vi "Tosca-Stream AI Data.vi"(0 "state in":T1, 5 "Data":cluster{dbl[][], bool[][]}, 11 "error in (no error)":errorcluster, 13 "stream":T2) -> (4 "state out":T1, 8 "filename":string, 15 "error out":errorcluster)   [LabVIEW 2020]
uses:
  Typedefs/Tosca-AI Stream Controls.ctl
  Typedefs/Tosca-AI Plot State.ctl
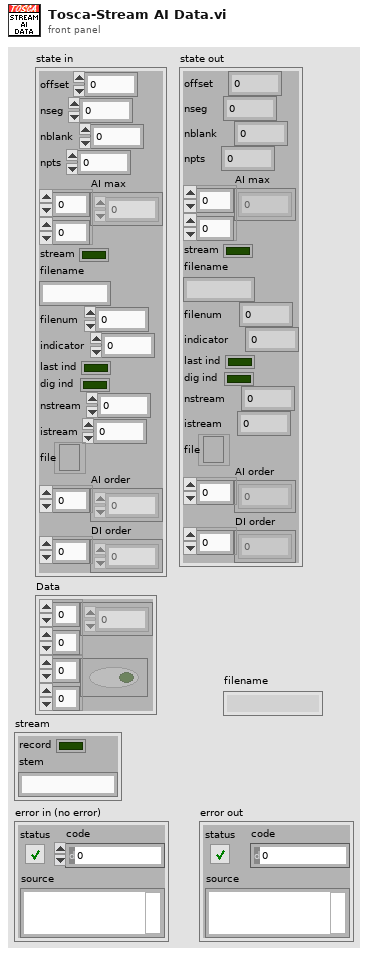
[diagram p1: front panel]
types:
  T1 = typedef "Tosca-AI Plot State.ctl" = cluster{"offset":i32, "nseg":i32, "nblank":i32, "npts":i32, "AI max":dbl[][], "stream":bool, "filename":string, "filenum":i32, "indicator":i32, "last ind":bool, "dig ind":bool, "nstream":i32, "istream":i32, "file":refnum<file>, "AI order":i32[], "DI order":i32[]}
  T2 = typedef "Tosca-AI Stream Controls.ctl" = cluster{"record":bool, "stem":string}
  T3 = enum16{"open", "replace", "create", "open or create", "replace or create", "replace or create with confirmation"}
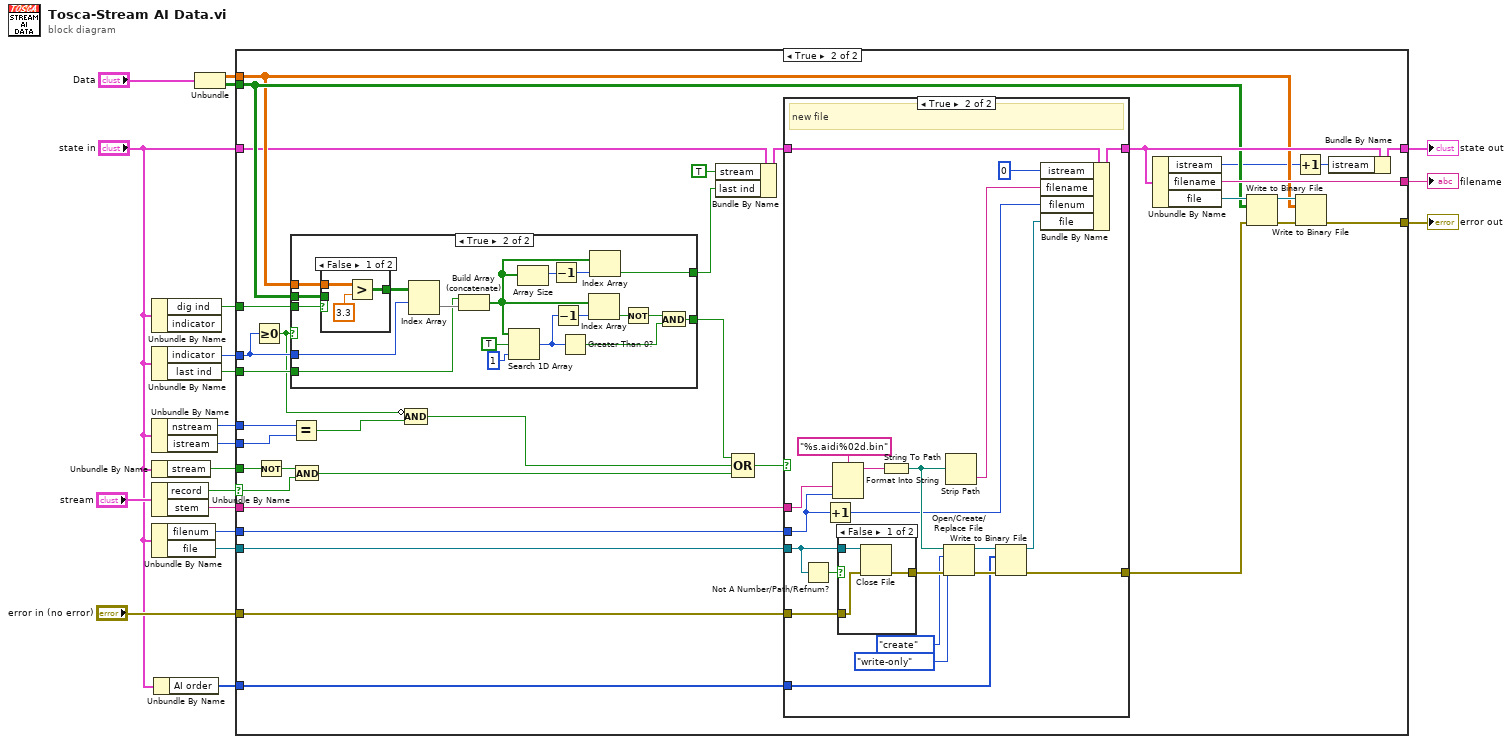
[diagram p0: block diagram]
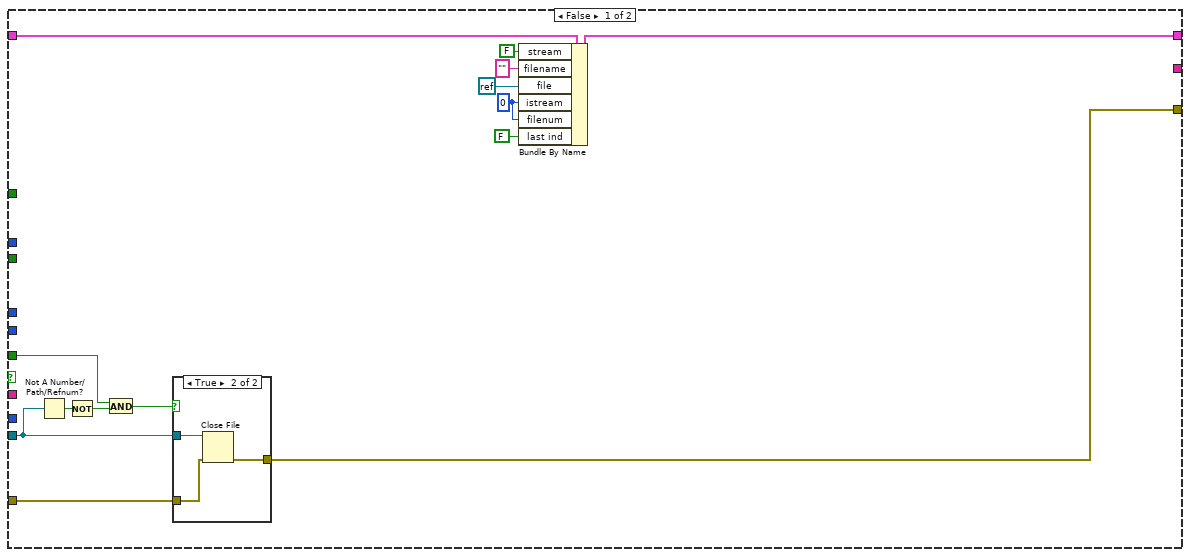
[diagram p2: hidden frame]
diagram:
  n1 = Unbundle By Name("state in") -> ("dig ind"=w18:bool)  [unwired: 1 out]
  n2 = Unbundle By Name("state in") -> ("indicator"=w11:i32, "last ind"=w12:bool)
  n3 = Unbundle By Name("state in") -> ("nstream"=w10:i32, "istream"=w9:i32)
  n4 = Unbundle By Name("state in") -> ("stream"=w13:bool)
  n5 = Unbundle By Name("stream") -> ("record"=w19:bool, "stem"=w17:string)
  n6 = Unbundle By Name("state in") -> ("filenum"=w6:i32, "file"=w8:refnum<file>)
  n7 = Unbundle By Name("state in") -> ("AI order"=w1:i32[])
  n8 = Unbundle("Data") -> (w15:dbl[][], w14:bool[][])
  n9 = case shown="True" w19 {
    selector: w19 -> [_ w68]
    tunnel: w18 -> [_ w72]
    tunnel: w17 -> [_ w73]
    tunnel: w15 -> [_ w48]
    tunnel: w14 -> [_ w52]
    tunnel: w11 -> [_ w71]
    tunnel: w13 -> [w29 w70]
    tunnel: w12 -> [_ w66]
    tunnel: w10 -> [_ w63]
    tunnel: w9 -> [_ w62]
    tunnel: w8 -> [w27 w60]
    tunnel: "state in" -> [w34 w46]
    tunnel: "error in (no error)" -> [w24 w59]
    tunnel: w6 -> [_ w58]
    tunnel: [w33 w44] -> w5
    tunnel: [_ w54] -> w4
    tunnel: [w23 w47] -> w3
    tunnel: w1 -> [_ w39]
    frame False {
      w22 = 0 ("istream")
      n10 = Not A Number/Path/Refnum?(number/path/refnum=w27) -> (NaN/Path/Refnum?=w31:bool)
      n11 = Not(x=w31) -> (.not. x?=w30:bool)
      n12 = And(x=w29, y=w30) -> (x .and. y?=w28:bool)
      n13 = case shown="True" w28 {
        tunnel: w27 -> [_ w38]
        tunnel: w24 -> [w35 w37]
        tunnel: [w35 w36] -> w23
        frame False {
        }
        frame True {
          n14 = Close File(refnum=w38, error in=w37) -> (error out=w36:errorcluster)  [unwired: 1 out]
        }
      }
      n15 = Bundle By Name(cluster=w34, "stream"=FALSE, "filename"="", "file"=refnum<k0> refnum, "istream"=w22, "filenum"=w22, "last ind"=FALSE) -> (w33:T1)
    }
    frame True {
      n16 = Greater Or Equal To 0?(x=w71) -> (x >= 0?=w40:bool)
      n17 = Not(x=w70) -> (.not. x?=w69:bool)
      n18 = case shown="True" w40 {
        tunnel: w72 -> [_ w92]
        tunnel: w71 -> [_ w88]
        tunnel: w52 -> [_ w91]
        tunnel: w48 -> [_ w90]
        tunnel: w66 -> [_ w85]
        tunnel: [_ w76] -> w64
        tunnel: [_ w74] -> w56
        frame False {
        }
        frame True {
          n19 = case shown="False" w92 {
            tunnel: w91 -> [_ w96]
            tunnel: w90 -> [w95 _]
            tunnel: [w93 w96] -> w89
            frame False {
              n20 = Greater?(x=w95, y=3.3) -> (0:w93:bool[][])
            }
            frame True {
            }
          }
          n21 = Index Array(array=w89, index (row)=w88) -> (element=w87:bool[])  [unwired: 1 in]
          n22 = Build Array (concatenate)(w85, w87) -> (w79:bool[])
          n23 = Search 1D Array(1D array=w79, element=TRUE, start index (0)=1) -> (index of element=w83:i32)
          n24 = Array Size(array=w79) -> (size(s)=w78:i32)
          n25 = Decrement(x=w78) -> (x-1=w77:i32)
          n26 = Decrement(x=w83) -> (x-1=w82:i32)
          n27 = Greater Than 0?(x=w83) -> (x > 0?=w80:bool)
          n28 = Index Array(array=w79, index=w82) -> (element=w81:bool)
          n29 = Index Array(array=w79, index=w77) -> (element=w74:bool)
          n30 = Not(x=w81) -> (.not. x?=w75:bool)
          n31 = And(x=w75, y=w80) -> (x .and. y?=w76:bool)
        }
      }
      n32 = Equal?(x=w63, y=w62) -> (x = y?=w61:bool)
      n33 = And(x=w69, y=w68) -> (x .and. y?=w67:bool)
      n34 = Compound Arithmetic op=AND(invert w40, w61) -> (w41:bool)
      n35 = Bundle By Name(cluster=w46, "stream"=TRUE, "last ind"=w56) -> (w57:T1)
      n36 = Compound Arithmetic op=OR(w64, w41, w67) -> (w65:bool)
      n37 = case shown="True" w65 {
        tunnel: w73 -> [_ w115]
        tunnel: w60 -> [_ w118]
        tunnel: w59 -> [w97 w117]
        tunnel: w58 -> [_ w114]
        tunnel: [w97 w100] -> w49
        tunnel: w57 -> [w98 w108]
        tunnel: [w98 w107] -> w55
        tunnel: w39 -> [_ w99]
        frame False {
        }
        frame True {
          # "new file"
          n38 = Not A Number/Path/Refnum?(number/path/refnum=w118) -> (NaN/Path/Refnum?=w119:bool)
          n39 = Increment(x=w114) -> (x+1=w105:i32)
          n40 = Format Into String(format string="%s.aidi%02d.bin", w115, w114) -> (resulting string=w113:string)  [unwired: 2 in, 1 out]
          n41 = case shown="False" w119 {
            tunnel: w118 -> [w122 _]
            tunnel: w117 -> [w121 w123]
            tunnel: [w120 w123] -> w111
            frame False {
              n42 = Close File(refnum=w122, error in=w121) -> (error out=w120:errorcluster)  [unwired: 1 out]
            }
            frame True {
            }
          }
          n43 = String To Path(string=w113) -> (path=w112:path)
          n44 = Open/Create/Replace File(file path (use dialog)=w112, error in=w111, operation (0:open)=T3."create", access (0:read/write)=enum16{"read/write", "read-only", "write-only"}."write-only") -> (refnum out=w102:refnum<file>, error out=w103:errorcluster)  [unwired: 2 in, 1 out]
          n45 = Strip Path(path=w112) -> (name=w106:string)  [unwired: 1 out]
          n46 = Write to Binary File(file (use dialog)=w102, data=w99, error in=w103) -> (refnum out=w101:refnum<file>, error out=w100:errorcluster)  [unwired: 3 in, 1 out]
          n47 = Bundle By Name(cluster=w108, "istream"=0, "filename"=w106, "filenum"=w105, "file"=w101) -> (w107:T1)
        }
      }
      n48 = Unbundle By Name(w55) -> ("istream"=w42:i32, "filename"=w54:string, "file"=w53:refnum<file>)
      n49 = Write to Binary File(file (use dialog)=w53, data=w52, error in=w49) -> (refnum out=w51:refnum<file>, error out=w50:errorcluster)  [unwired: 3 in, 1 out]
      n50 = Increment(x=w42) -> (x+1=w43:i32)
      n51 = Write to Binary File(file (use dialog)=w51, data=w48, error in=w50) -> (error out=w47:errorcluster)  [unwired: 3 in, 2 out]
      n52 = Bundle By Name(cluster=w55, "istream"=w43) -> (w44:T1)
    }
  }
  "error out" <- w3
  "state out" <- w5
  "filename" <- w4
